vi "Set Enable State on Multiple Controls.vi"(8 "启用？":bool, 11 "数组":refnum<vi>[](array[refnum])) -> ()   [LabVIEW 2022 SP3]
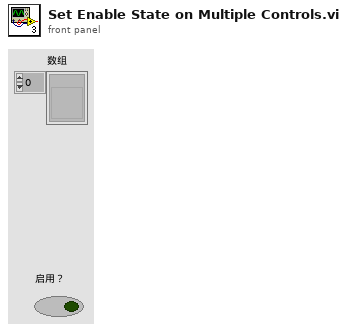
[diagram p1: front panel]
types:
  T1 = enum16{"Enabled", "Disabled", "Disabled and Grayed Out"}
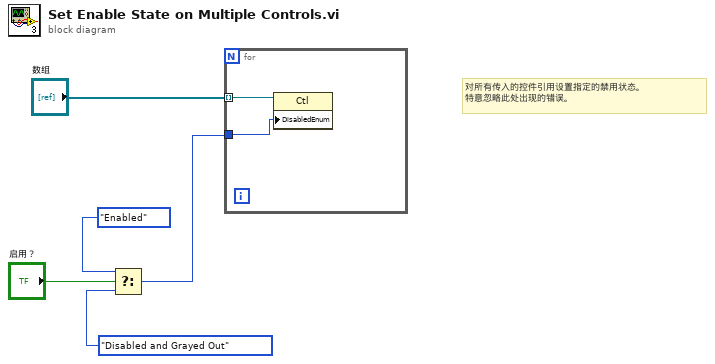
[diagram p0: block diagram]
diagram:
  # "对所有传入的控件引用设置指定的禁用状态。\n特意忽略此处出现的错误。"
  n1 = Select(t=T1."Enabled", s="启用？", f=T1."Disabled and Grayed Out") -> (s? t:f=w1:T1)
  n2 = for {
    tunnel: "数组" -> [w7] mode=indexing
    tunnel: w1 -> [w6]
    n3 = property class="Ctl"(reference=w7, "DisabledEnum"=w6) -> ()  [unwired: 1 in, 2 out]
  }
